vi "E19_MáquinaDeEstados.vi"() -> ()   [LabVIEW 2026]
panel:
  out "String":string="Paso 3"
  in  "stop":bool
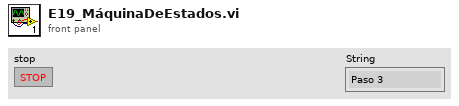
[diagram p1: front panel]
types:
  T1 = enum16{"Inicio", "Paso 1", "Paso 2", "Paso 3", "Finalizar"}
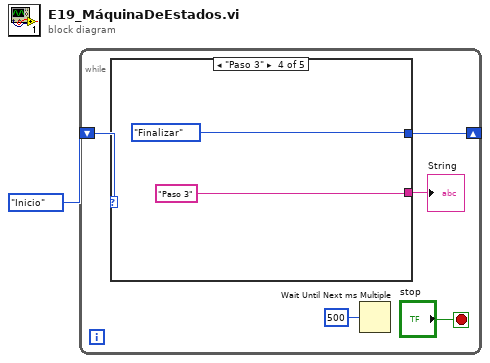
[diagram p0: block diagram]
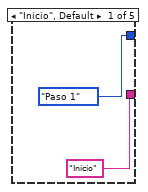
[diagram p2: hidden frame]
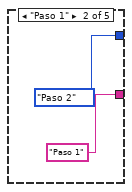
[diagram p3: hidden frame]
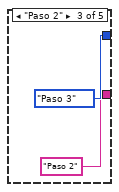
[diagram p4: hidden frame]
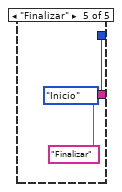
[diagram p5: hidden frame]
diagram:
  n1 = while {
    shift-right: [w4] -> _
    shift-left: T1."Inicio" -> [w5]
    stop <- "stop" stop-if-true
    n2 = case shown="\"Paso 3\"" w5 {
      tunnel: [T1."Paso 1" T1."Paso 2" T1."Paso 3" T1."Finalizar" T1."Inicio"] -> w4
      tunnel: ["Inicio" "Paso 1" "Paso 2" "Paso 3" "Finalizar"] -> w3
      frame "Inicio", Default {
      }
      frame "Paso 1" {
      }
      frame "Paso 2" {
      }
      frame "Paso 3" {
      }
      frame "Finalizar" {
      }
    }
    "String" <- w3
    n3 = Wait Until Next ms Multiple(millisecond multiple=u32 500) -> ()  [unwired: 1 out]
  }
